vi "Actor Core.vi"(8 "error in":errorcluster caption="错误输入", 11 "GlobalPlanner in":refnum<class "GlobalPlanner.lvclass"> caption="操作者输入") -> (0 "error out":errorcluster caption="错误输出", 3 "Actor out":refnum<class "Actor.lvclass"> caption="操作者输出")   [LabVIEW 2014, in "GlobalPlanner.lvlib" / "GlobalPlanner.lvclass"]
doc: "(<B>文件名</B>：Actor Framework.lvlib:Actor.lvclass:Actor Core.vi)\n\n接收发送至操作者的消息，响应消息并处理可能导致操作者关闭的错误。\n\n子孙类重写该VI，使操作者完成特定的任务。使用调用父方法节点实现重写。"
uses:
  GlobalPlanner.lvclass
  <vilib>/ActorFramework/Actor/Actor.lvclass
  ctl/Semantic_Voice_Array.ctl
  <vilib>/ActorFramework/Actor/Actor.lvclass/Actor.ctl
  GlobalPlanner.lvclass/GlobalPlanner.ctl
  <vilib>/ActorFramework/Message Enqueuer/Message Enqueuer.lvclass/Message Enqueuer.ctl
  <vilib>/ActorFramework/Message Enqueuer/Enqueue.vi
  Global_var/Global_var.vi
  <vilib>/ActorFramework/Message Priority Queue/Priority Enqueue.vi
  Wrapper_lib/zsActor/ActorWrapper.lvclass
  Voice_lib/VoiceControl/Voice.lvclass
panel:
  out "GlobalPlanner_Recycle":bool
  out "Semantic_Voice_Array":T1
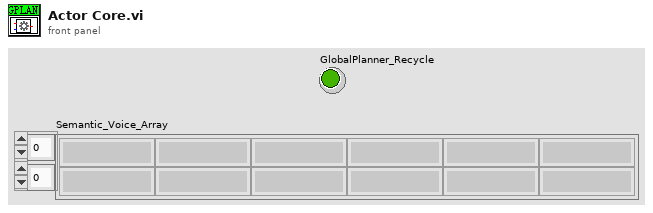
[diagram p1: front panel]
types:
  T1 = typedef "Semantic_Voice_Array.ctl" = string[][]
  T2 = cluster{"now_pose_X":dbl, "now_pose_Y":dbl, "now_pose_Rot_deg":dbl}
  T3 = cluster{"起点":string, "终点":string, "动作":string, "方向":string, "距离":string, "速度":string}
  T4 = typedef "Point.ctl" = cluster{"x":dbl, "y":dbl, "z":dbl}
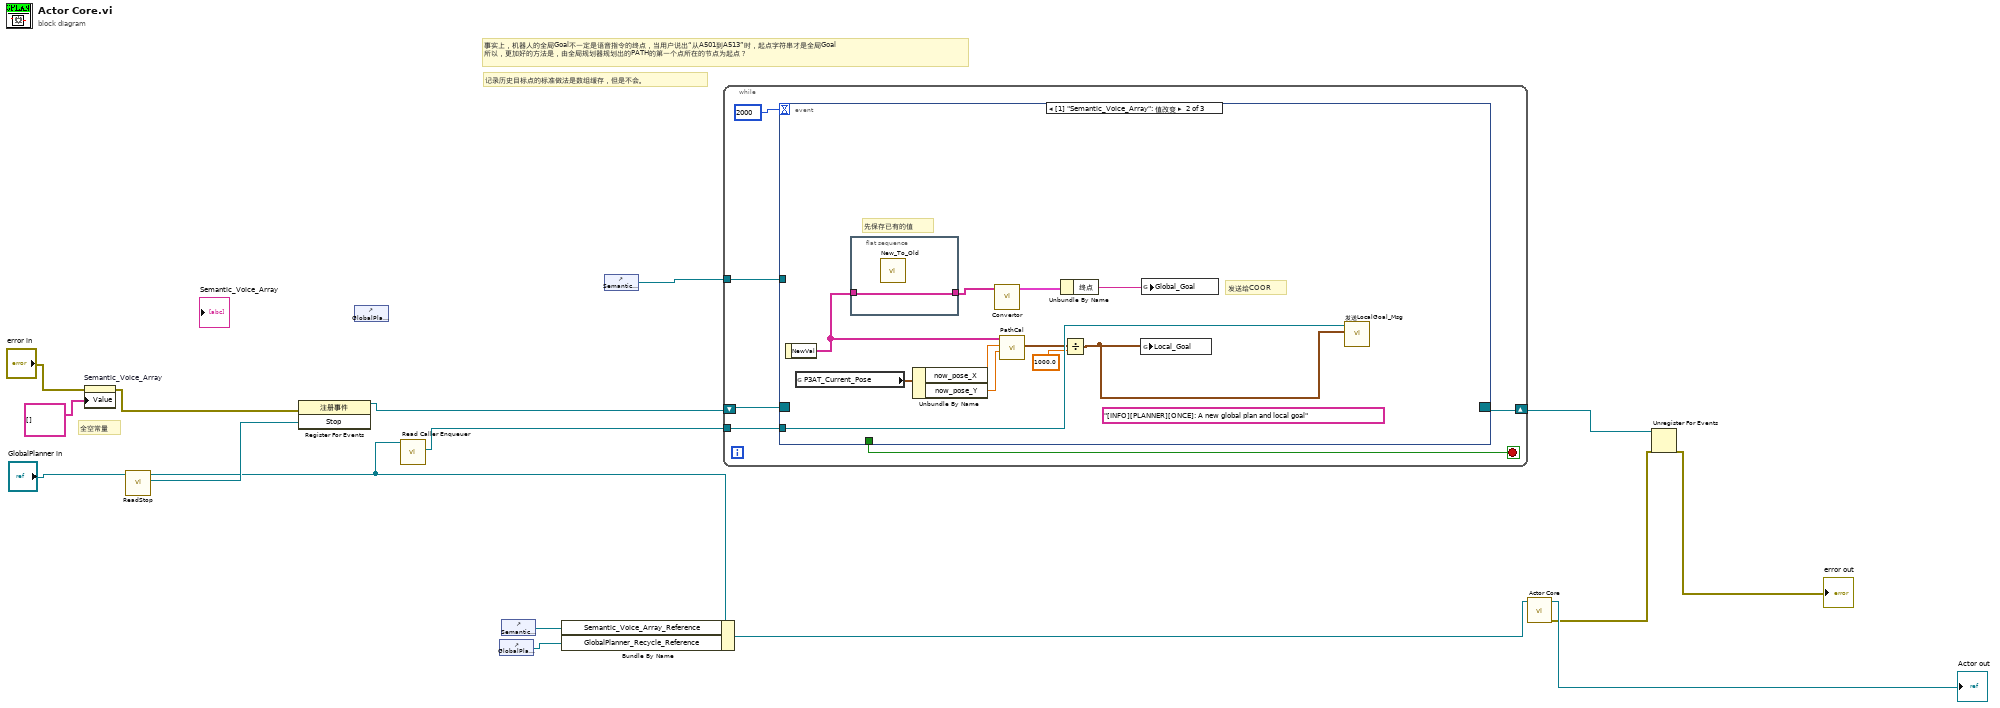
[diagram p0: block diagram]
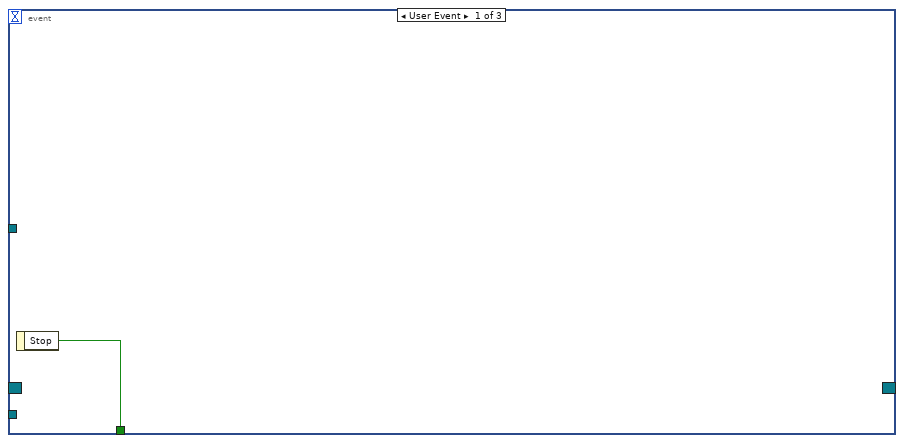
[diagram p2: hidden frame]
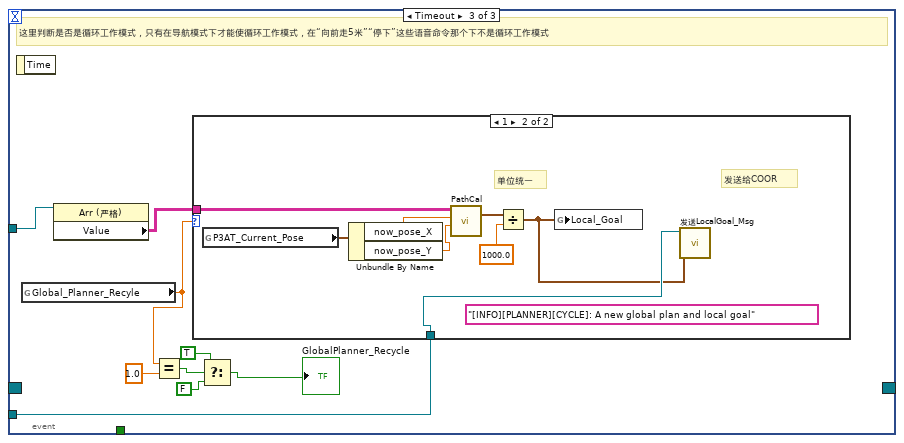
[diagram p3: hidden frame]
diagram:
  # "记录历史目标点的标准做法是数组缓存，但是不会。"
  # "事实上，机器人的全局Goal不一定是语音指令的终点，当用户说出“从A501到A513”时，起点字符串才是全局Goal\n所以，更加好的方法是，由全局规划器规划出的PATH的第一个点所在的节点为起点？"
  # "全空常量"
  n1 = property on="Semantic_Voice_Array" class="Arr (严格)"(error in="error in", "Value"=T1 [] ("Semantic_Voice_Array 2")) -> (error out=w12:errorcluster)  [unwired: 1 in, 1 out]
  n2 = call-dynamic "ReadStop.vi"("zsActor输入"="GlobalPlanner in") -> ("Stop"=w14:refnum<user-event>, "zsActor输出"=w8:refnum<class "GlobalPlanner.lvclass">)  [unwired: 8 in, 1 out]
  n3 = register-events(error in=w12, w14) -> (reference out=w6:refnum<event-registration>)  [unwired: 1 in, 1 out]
  n4 = control-ref of="GlobalPlanner_Recycle"() -> ()  [unwired: 1 out]
  n5 = call <vilib>:"Read Caller Enqueuer.vi"("Actor"=w8) -> ("Caller Enqueuer"=w7:refnum<class "Message Enqueuer.lvclass">)  [unwired: 10 in]
  n6 = control-ref of="GlobalPlanner_Recycle"() -> (w1:refnum<vi>)
  n7 = control-ref of="Semantic_Voice_Array"() -> (w10:refnum<vi>)
  n8 = Bundle By Name(cluster=w8, "Semantic_Voice_Array_Reference"=w10, "GlobalPlanner_Recycle_Reference"=w1) -> (w9:refnum<class "GlobalPlanner.lvclass">)
  n9 = control-ref of="Semantic_Voice_Array"() -> (w2:refnum<vi>)
  n10 = while {
    tunnel: w7 -> [w22]
    shift-right: [w20] -> w5
    shift-left: w6 -> [w21]
    tunnel: w2 -> [w17]
    stop <- w19 stop-if-true
    n11 = event shown="[1] \"Semantic_Voice_Array\": 值改变" {
      selector: w21 -> [_ _ _]
      dyn-events: [_ _ _] -> w20
      timeout: 2000 -> [_ _ _]
      tunnel: w22 -> [_ w27 w42]
      tunnel: [w23 _ _] -> w19
      tunnel: w17 -> [_ _ w44]
      event User Event {
        n12 = event-data() -> ("Stop"=w23:bool)  [unwired: 1 in]
      }
      event Value Change {
        (unwired) "[INFO][PLANNER][ONCE]: A new global plan and local goal" ("Event Text")
        # "发送给COOR"
        # "先保存已有的值"
        n13 = event-data() -> ("NewVal"=w30:T1)  [unwired: 1 in]
        n14 = global read "Global_var.vi" "P3AT_Current_Pose"() -> (w34:T2)
        n15 = flat-sequence {
          tunnel: w30 -> [w35]
          tunnel: [w35] -> w29
          frame #0 {
            n16 = call "New_To_Old.vi"() -> ()  [unwired: 11 in, 1 out]
          }
        }
        n17 = Unbundle By Name(w34) -> ("now_pose_X"=w33:dbl, "now_pose_Y"=w32:dbl)
        n18 = call "Convertor.vi"("机器人指令数组"=w29) -> ("机器人语音指令数据簇"=w31:T3)  [unwired: 10 in]
        n19 = call "PathCal.vi"("pose_y"=w32, "pose_x"=w33, "语音命令数组"=w30) -> ("Local_Goal"=w26:T4)  [unwired: 7 in, 1 out]
        n20 = Unbundle By Name(w31) -> ("终点"=w28:string)
        n21 = Divide(x=w26, y=1000.0) -> (x/y=w24:T4)
        n22 = global write "Global_var.vi" "Local_Goal"(w24) -> ()
        n23 = global write "Global_var.vi" "Global_Goal"(w28) -> ()
        n24 = call "发送LocalGoal_Msg.vi"("值(信号)"=w24, "消息待入队列"=w27) -> ()  [unwired: 8 in, 2 out]
      }
      event Timeout {
        # "这里判断是否是循环工作模式，只有在导航模式下才能使循环工作模式，在“向前走5米”“停下”这些语音命令那个下不是循环工作模式"
        n25 = event-data() -> ()  [unwired: 1 in, 1 out]
        n26 = global read "Global_var.vi" "Global_Planner_Recyle"() -> (w41:dbl)
        n27 = property class="Arr (严格)"(reference=w44) -> ("Value"=w43:T1)  [unwired: 1 in, 2 out]
        n28 = Equal?(x=w41, y=1.0) -> (x = y?=w39:bool)
        n29 = case shown="1" w41 {
          tunnel: w43 -> [_ w49]
          tunnel: w42 -> [_ w48]
          frame 0, Default {
          }
          frame 1 {
            (unwired) "[INFO][PLANNER][CYCLE]: A new global plan and local goal" ("Event Text")
            # "单位统一"
            # "发送给COOR"
            n30 = global read "Global_var.vi" "P3AT_Current_Pose"() -> (w52:T2)
            n31 = Unbundle By Name(w52) -> ("now_pose_X"=w51:dbl, "now_pose_Y"=w50:dbl)
            n32 = call "PathCal.vi"("pose_y"=w50, "pose_x"=w51, "语音命令数组"=w49) -> ("Local_Goal"=w47:T4)  [unwired: 7 in, 1 out]
            n33 = Divide(x=w47, y=1000.0) -> (x/y=w46:T4)
            n34 = global write "Global_var.vi" "Local_Goal"(w46) -> ()
            n35 = call "发送LocalGoal_Msg.vi"("值(信号)"=w46, "消息待入队列"=w48) -> ()  [unwired: 8 in, 2 out]
          }
        }
        n36 = Select(t=TRUE, s=w39, f=FALSE) -> (s? t:f=→"GlobalPlanner_Recycle":bool)
      }
    }
  }
  n37 = call-parent "Actor Core.vi"("Actor in"=w9) -> ("error out"=w4:errorcluster, "Actor out"=→"Actor out":refnum<class "Actor.lvclass">)  [unwired: 9 in]
  n38 = Unregister For Events(event registration refnum=w5, error in=w4) -> (error out=→"error out":errorcluster)
